vi "Read Number.vi"(8 "error in (no error)":errorcluster, 11 "Example in":refnum<class "Example.lvclass">) -> (0 "error out":errorcluster, 2 "Number":dbl, 3 "Example out":refnum<class "Example.lvclass">)   [LabVIEW 2012, in "CS++Core-Examples.lvlib" / "Example.lvclass"]
doc: "Read number"
uses:
  Example.lvclass
  Example.lvclass/Example.ctl
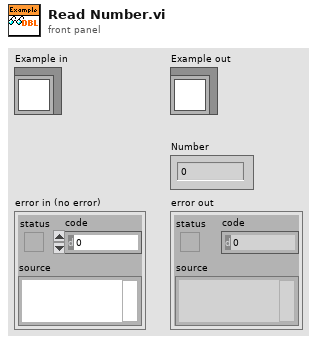
[diagram p1: front panel]
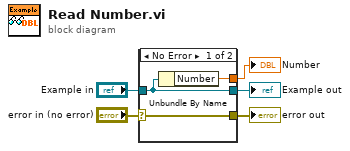
[diagram p0: block diagram]
diagram:
  n1 = case shown="No Error" "error in (no error)" {
    selector: "error in (no error)" -> [w8 w9]
    tunnel: [w8 w9] -> w4
    tunnel: [w7 w10] -> w2
    tunnel: "Example in" -> [w7 w10]
    tunnel: [w6 _] -> w1
    frame No Error {
      n2 = Unbundle By Name(w7) -> ("Number"=w6:dbl)
    }
    frame Error {
    }
  }
  "error out" <- w4
  "Example out" <- w2
  "Number" <- w1
